vi "基础12.vi"() -> ()   [LabVIEW 2014]
panel:
  out "数值 2":dbl
  in  "数值":dbl
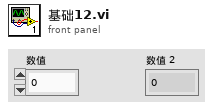
[diagram p1: front panel]
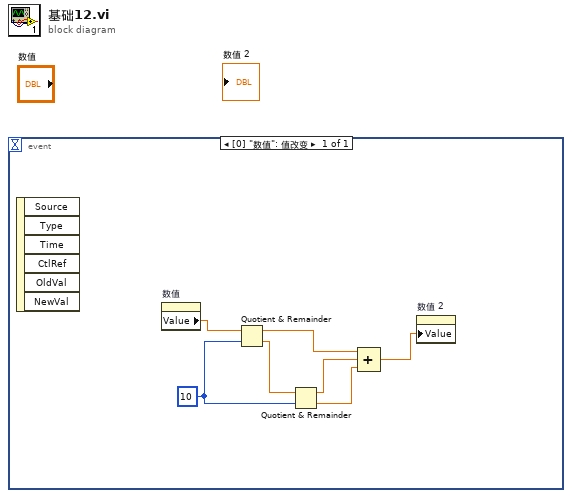
[diagram p0: block diagram]
diagram:
  n1 = event shown="[0] \"数值\": 值改变" {
    selector: _ -> [_]
    dyn-events: _ -> [_]
    timeout: _ -> [_]
    event "数值": Value Change {
      w5 = 10
      n2 = event-data() -> ()  [unwired: 1 in, 6 out]
      n3 = property on="数值" class="DigNum (严格)"() -> ("Value"=w7:dbl)  [unwired: 2 in, 2 out]
      n4 = Quotient & Remainder(x=w7, y=w5) -> (x-y*floor(x/y)=w4:dbl, floor(x/y)=w6:dbl)
      n5 = Quotient & Remainder(x=w6, y=w5) -> (x-y*floor(x/y)=w3:dbl, floor(x/y)=w2:dbl)
      n6 = Compound Arithmetic op=ADD(w4, w3, w2) -> (w1:dbl)
      n7 = property on="数值 2" class="DigNum (严格)"("Value"=w1) -> ()  [unwired: 2 in, 2 out]
    }
  }
